vi "PID Advanced.vi"   [LabVIEW 2020, in "NI_PID_pid.lvlib"]
doc: "Implements a PID controller using a PID algorithm with advanced optional features. The advanced PID algorithm includes the features of the algorithm the PID VI uses, as well as manual mode control with bumpless manual-to-automatic transitions, nonlinear integral action, two degree-of-freedom control, and error-squared control. Use the DBL instance of this VI to implement a single control loop. Use the DBL Array instance to implement parallel multi-loop control."
uses:
  NI_PID_pid.lvlib
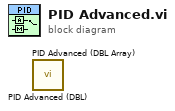
[diagram p0: block diagram]
diagram:
  n1 = call "PID Advanced (DBL).vi"() -> ()  [unwired: 14 in, 2 out]
  n2 = call "PID Advanced (DBL Array).vi"() -> ()  [unwired: 14 in, 2 out]
